vi "StratifiedKFold.vi"(6 "Groups":string[][](array[string]), 8 "error in (no error)":errorcluster caption="entrée d'erreur (pas d'erreur)", 9 "y":string[][](array[string]), 10 "X":string[][](array[string]), 11 "StratifiedKFold":T2={"n_splits"=5, "shuffle"=FALSE, "random_state"=-1} {"random_state" min=-1}) -> (0 "error out":errorcluster caption="sortie d'erreur", 3 "Split":T1(array[cluster]))   [LabVIEW 2020]
doc: "Stratified K-Folds cross-validator\n\nProvides train/test indices to split data in train/test sets.\n\nThis cross-validation object is a variation of KFold that returns stratified folds. The folds are made by preserving the percentage of samples for each class.\n\n\n\nParameters :\n\n- n_splits : int, default=5\nNumber of folds. Must be at least 2.\n\n- shuffle : bool, default=False\nWhether to shuffle each class’s samples before splitting into batches. Note that the samples within each split will not be shuffled.\n\n- random_state : int or RandomState instance, default=None=-1\nWhen shuffle is True, random_state affects the ordering of the indices, which controls the randomness of each fold for each class. Otherwise, leave random_state as None. Pass an int for reproducible output across multiple function calls. \n\n\nMethods : Split\n\nGenerate indices to split data into training and test set.\n\nParameters : \n\n- X : array-like of shape (n_samples, n_features)\nTraining data, where n_samples is the number of samples and n_features is the number of features.\n\nNote that providing y is sufficient to generate the splits and hence np.zeros(n_samples) may be used as a placeholder for X instead of actual training data.\n\n- y : array-like of shape (n_samples,)\nThe target variable for supervised learning problems. Stratification is done based on the y labels.\n\n- groups : object\nAlways ignored, exists for compatibility.\n\nYields : \n\n- train : ndarray\nThe training set indices for that split.\n\n- test : ndarray\nThe testing set indices for that split."
uses:
  StratifiedKFold.lvclass
panel:
  out "StratifiedKFold.lvclass":refnum<class "StratifiedKFold.lvclass">
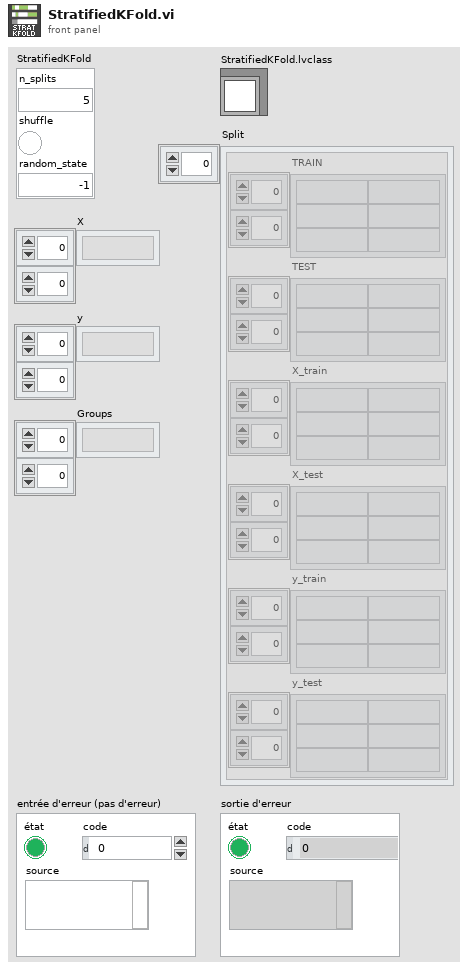
[diagram p1: front panel]
types:
  T1 = cluster{"TRAIN":string[][], "TEST":string[][], "X_train":string[][], "X_test":string[][], "y_train":string[][], "y_test":string[][]}[]
  T2 = cluster{"n_splits":i32, "shuffle":bool, "random_state":i32}
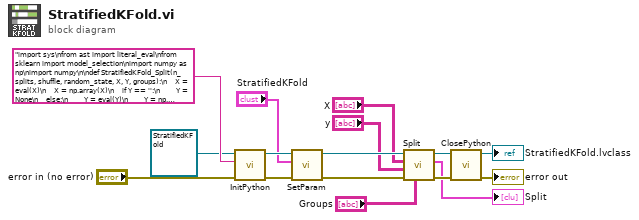
[diagram p0: block diagram]
diagram:
  n1 = call-dynamic "InitPython.vi"("error in (no error)"="error in (no error)", "Python Instruction"="import sys\nfrom ast import literal_eval\nfrom sklearn import model_selection\nimport numpy as np\nimport numpy\n\ndef StratifiedKFold_Split(n_splits, shuffle, random_state, X, Y, groups):\n    X = eval(X)\n    X = np.array(X)\n    if Y == '':\n        Y = None\n    else:\n        Y = eval(Y)\n        Y = np.array(Y)\n    if groups == '':\n        groups = None\n    else:\n        groups = eval(groups)\n        groups = np.array(groups)\n    if random_state == -1:\n        random_state = None\n    list_return = []\n    try:\n        for train_index, test_index in model_selection.StratifiedKFold(n_splits, shuffle, random_state).split(X, Y, groups):\n            list_return = list_return +[\"TRAIN:\", train_index.tolist(), \"TEST:\", test_index.tolist()]\n            X_train, X_test = X[train_index].tolist(), X[test_index].tolist()\n            y_train, y_test = Y[train_index].tolist(), Y[test_index].tolist()\n            list_return = list_return +[\"X_train:\", X_train, \"X_test:\", X_test, \"y_train:\", y_train, \"y_test:\", y_test]\n        return str(list_return)\n    except:\n        erreur = sys.exc_info()\n        typerr = u\"%s\" % (erreur[0])\n        typerr = typerr[typerr.find(\"'\")+1:typerr.rfind(\"'\")]\n        msgerr = u\"%s\" % (erreur[1])\n        message = str('/!\\\\ {0} : {1}'. format(typerr,msgerr))\n        return message", "Scikit-learn en entrée"=refnum<class "StratifiedKFold.lvclass"> refnum ("StratifiedKFold.lvclass")) -> ("error out"=w13:errorcluster, "Scikit-learn en sortie"=w12:refnum<class "StratifiedKFold.lvclass">)  [unwired: 7 in]
  n2 = call-dynamic "SetParam.vi"("error in (no error)"=w13, "StratifiedKFold"="StratifiedKFold", "StratifiedKFold.lvclass"=w12) -> ("error out"=w9:errorcluster, "StratifiedKFold.lvclass"=w10:refnum<class "StratifiedKFold.lvclass">)  [unwired: 7 in]
  n3 = call-dynamic "Split.vi"("Groups"="Groups", "error in (no error)"=w9, "y"="y", "X"="X", "StratifiedKFold.lvclass"=w10) -> ("error out"=w8:errorcluster, "Split"=→"Split":T1, "StratifiedKFold.lvclass"=w7:refnum<class "StratifiedKFold.lvclass">)  [unwired: 4 in]
  n4 = call-dynamic "ClosePython.vi"("error in (no error)"=w8, "Scikit-learn en entrée"=w7) -> ("error out"=→"error out":errorcluster, "Scikit-learn en sortie"=→"StratifiedKFold.lvclass":refnum<class "StratifiedKFold.lvclass">)  [unwired: 8 in]
